vi "Parse Data INSPVAX(SubVI).vi"(11 "Parse Data Array":string[](array[string])=["37.37010082408", "126.72084278410", "9.8363", "22.3000", "-0.0077", "0.0002", "0.0002", "-0.786930858", "0.220983047", "80.255496235", "0.2109", "0.1616", "0.2842", "0.0344", "0.0343", "0.0312", "0.0727", "0.0733", "4.8905", "0f000005", "0*84218c18\n\t"]) -> (3 "output cluster":T1={"Latitude"={"Valid?"=TRUE, "Latitude (Deg)"=37.37010082408}, "Longitude"={"Valid?"=TRUE, "Longitude (Deg)"=126.7208427841}, "Height"={"Valid?"=TRUE, "Height (m)"=9.8363}, "Undulation"={"Valid?"=TRUE, "Undulation(m)"=22.3}, "North Vel"={"Valid?"=TRUE, "North Vel (m/s)"=-0.0077}, "East Vel"={"Valid?"=TRUE, "East Vel (m/s)"=0.0002}, "Up Vel"={"Valid?"=TRUE, "Up Vel (m/s)"=0.0002}, "Roll"={"Valid?"=TRUE, "Roll (degrees)"=-0.786930858}, "Pitch"={"Valid?"=TRUE, "Pitch (degrees)"=0.220983047}, "Azimuth"={"Valid?"=TRUE, "Azimuth (degrees)"=80.255496235}, "Lat deviation"={"Valid?"=TRUE, "Lat deviation (m)"=0.2109}, "Long deviation"={"Valid?"=TRUE, "Long deviation (m)"=0.1616}, "Height deviation"={"Valid?"=TRUE, "Height deviation (m)"=0.2842}, "North vel deviation"={"Valid?"=TRUE, "North vel deviation (m/s)"=0.0344}, "East vel deviation"={"Valid?"=TRUE, "East vel deviation (m/s)"=0.0343}, "Up vel deviation"={"Valid?"=TRUE, "Up vel deviation (m/s)"=0.0312}, "Roll deviation"={"Valid?"=TRUE, "Roll deviation (degrees)"=0.0727}, "Pitch deviation"={"Valid?"=TRUE, "Pitch deviation (degrees)"=0.0733}, "Azimuth deviation"={"Valid?"=TRUE, "Azimuth deviation (degrees)"=4.8905}, "Ext sol status"={"Valid?"=TRUE, "Ext sol status"=0.0}})   [LabVIEW 2019]
panel:
  out "x = y?":bool=TRUE
  out "size":i32=21
  out "output cluster 2":T1={"Latitude"={"Valid?"=TRUE, "Latitude (Deg)"=37.37010082408}, "Longitude"={"Valid?"=TRUE, "Longitude (Deg)"=126.7208427841}, "Height"={"Valid?"=TRUE, "Height (m)"=9.8363}, "Undulation"={"Valid?"=TRUE, "Undulation(m)"=22.3}, "North Vel"={"Valid?"=TRUE, "North Vel (m/s)"=-0.0077}, "East Vel"={"Valid?"=TRUE, "East Vel (m/s)"=0.0002}, "Up Vel"={"Valid?"=TRUE, "Up Vel (m/s)"=0.0002}, "Roll"={"Valid?"=TRUE, "Roll (degrees)"=-0.786930858}, "Pitch"={"Valid?"=TRUE, "Pitch (degrees)"=0.220983047}, "Azimuth"={"Valid?"=TRUE, "Azimuth (degrees)"=80.255496235}, "Lat deviation"={"Valid?"=TRUE, "Lat deviation (m)"=0.2109}, "Long deviation"={"Valid?"=TRUE, "Long deviation (m)"=0.1616}, "Height deviation"={"Valid?"=TRUE, "Height deviation (m)"=0.2842}, "North vel deviation"={"Valid?"=TRUE, "North vel deviation (m/s)"=0.0344}, "East vel deviation"={"Valid?"=TRUE, "East vel deviation (m/s)"=0.0343}, "Up vel deviation"={"Valid?"=TRUE, "Up vel deviation (m/s)"=0.0312}, "Roll deviation"={"Valid?"=TRUE, "Roll deviation (degrees)"=0.0727}, "Pitch deviation"={"Valid?"=TRUE, "Pitch deviation (degrees)"=0.0733}, "Azimuth deviation"={"Valid?"=TRUE, "Azimuth deviation (degrees)"=4.8905}, "Ext sol status"={"Valid?"=TRUE, "Ext sol status"=0.0}}
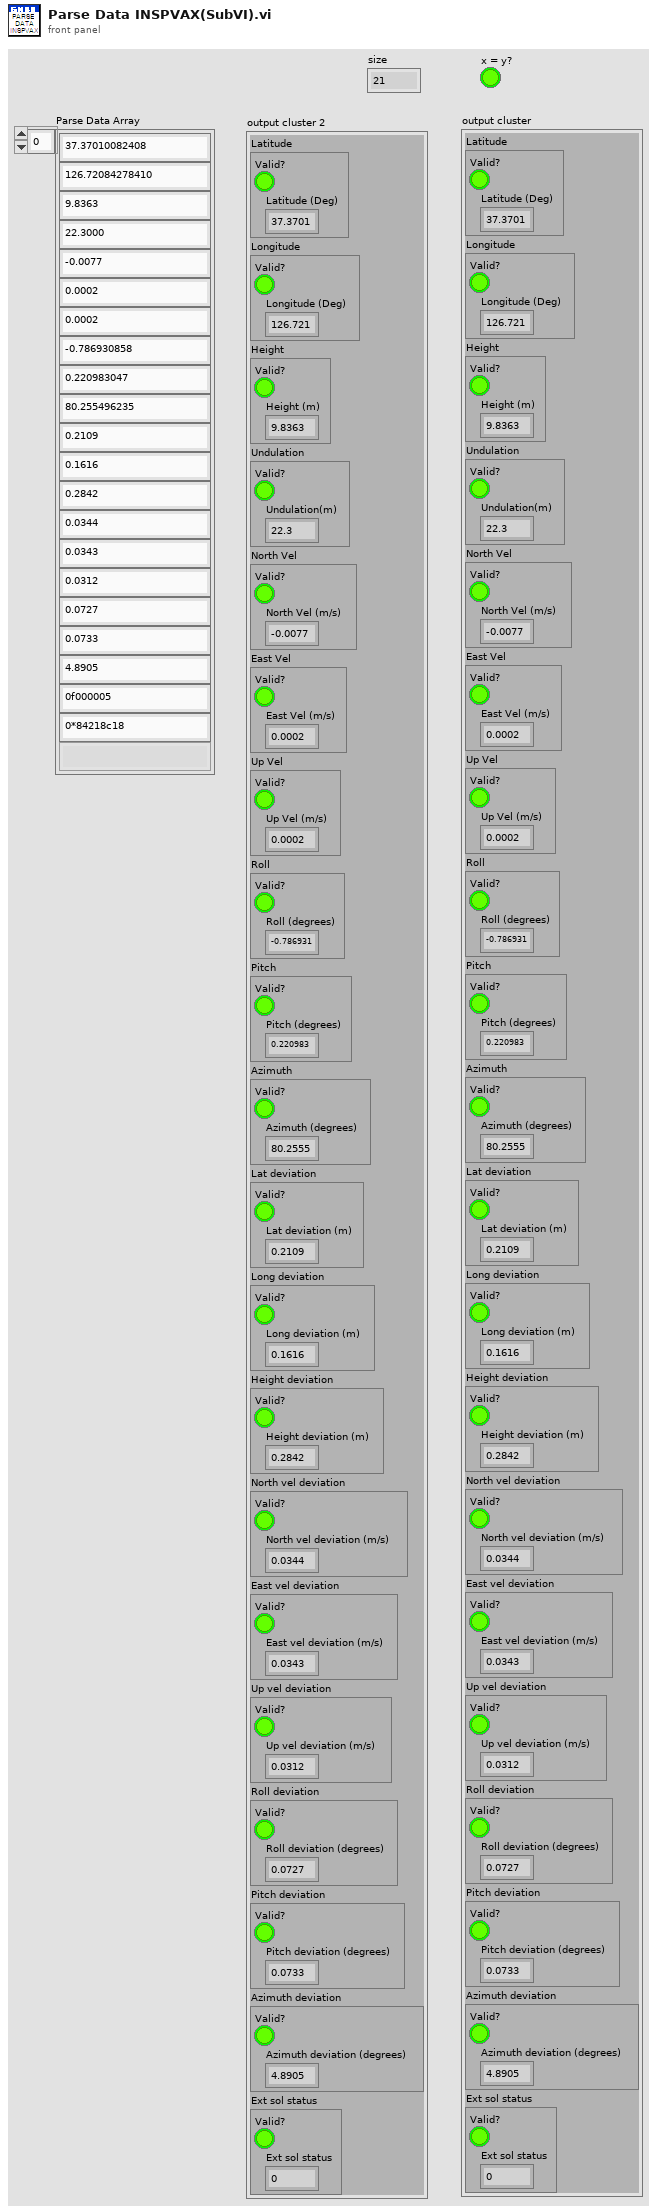
[diagram p1: front panel]
types:
  T1 = cluster{"Latitude":cluster{"Valid?":bool, "Latitude (Deg)":dbl}, "Longitude":cluster{"Valid?":bool, "Longitude (Deg)":dbl}, "Height":cluster{"Valid?":bool, "Height (m)":dbl}, "Undulation":cluster{"Valid?":bool, "Undulation(m)":dbl}, "North Vel":cluster{"Valid?":bool, "North Vel (m/s)":dbl}, "East Vel":cluster{"Valid?":bool, "East Vel (m/s)":dbl}, "Up Vel":cluster{"Valid?":bool, "Up Vel (m/s)":dbl}, "Roll":cluster{"Valid?":bool, "Roll (degrees)":dbl}, "Pitch":cluster{"Valid?":bool, "Pitch (degrees)":dbl}, "Azimuth":cluster{"Valid?":bool, "Azimuth (degrees)":dbl}, "Lat deviation":cluster{"Valid?":bool, "Lat deviation (m)":dbl}, "Long deviation":cluster{"Valid?":bool, "Long deviation (m)":dbl}, "Height deviation":cluster{"Valid?":bool, "Height deviation (m)":dbl}, "North vel deviation":cluster{"Valid?":bool, "North vel deviation (m/s)":dbl}, "East vel deviation":cluster{"Valid?":bool, "East vel deviation (m/s)":dbl}, "Up vel deviation":cluster{"Valid?":bool, "Up vel deviation (m/s)":dbl}, "Roll deviation":cluster{"Valid?":bool, "Roll deviation (degrees)":dbl}, "Pitch deviation":cluster{"Valid?":bool, "Pitch deviation (degrees)":dbl}, "Azimuth deviation":cluster{"Valid?":bool, "Azimuth deviation (degrees)":dbl}, "Ext sol status":cluster{"Valid?":bool, "Ext sol status":dbl}}
  T2 = cluster{"Valid?":bool, "Pitch deviation (degrees)":dbl}
  T3 = cluster{"Valid?":bool, "Azimuth deviation (degrees)":dbl}
  T4 = cluster{"Valid?":bool, "Roll deviation (degrees)":dbl}
  T5 = cluster{"Valid?":bool, "Up vel deviation (m/s)":dbl}
  T6 = cluster{"Valid?":bool, "Height deviation (m)":dbl}
  T7 = cluster{"Valid?":bool, "North vel deviation (m/s)":dbl}
  T8 = cluster{"Valid?":bool, "East vel deviation (m/s)":dbl}
  T9 = cluster{"[0]":cluster{"Valid?":bool, "Latitude (Deg)":dbl}, "[1]":cluster{"Valid?":bool, "Latitude (Deg)":dbl}, "[2]":cluster{"Valid?":bool, "Latitude (Deg)":dbl}, "[3]":cluster{"Valid?":bool, "Latitude (Deg)":dbl}, "[4]":cluster{"Valid?":bool, "Latitude (Deg)":dbl}, "[5]":cluster{"Valid?":bool, "Latitude (Deg)":dbl}, "[6]":cluster{"Valid?":bool, "Latitude (Deg)":dbl}, "[7]":cluster{"Valid?":bool, "Latitude (Deg)":dbl}, "[8]":cluster{"Valid?":bool, "Latitude (Deg)":dbl}, "[9]":cluster{"Valid?":bool, "Latitude (Deg)":dbl}, "[10]":cluster{"Valid?":bool, "Latitude (Deg)":dbl}, "[11]":cluster{"Valid?":bool, "Latitude (Deg)":dbl}, "[12]":cluster{"Valid?":bool, "Latitude (Deg)":dbl}, "[13]":cluster{"Valid?":bool, "Latitude (Deg)":dbl}, "[14]":cluster{"Valid?":bool, "Latitude (Deg)":dbl}, "[15]":cluster{"Valid?":bool, "Latitude (Deg)":dbl}, "[16]":cluster{"Valid?":bool, "Latitude (Deg)":dbl}, "[17]":cluster{"Valid?":bool, "Latitude (Deg)":dbl}, "[18]":cluster{"Valid?":bool, "Latitude (Deg)":dbl}, "[19]":cluster{"Valid?":bool, "Latitude (Deg)":dbl}}
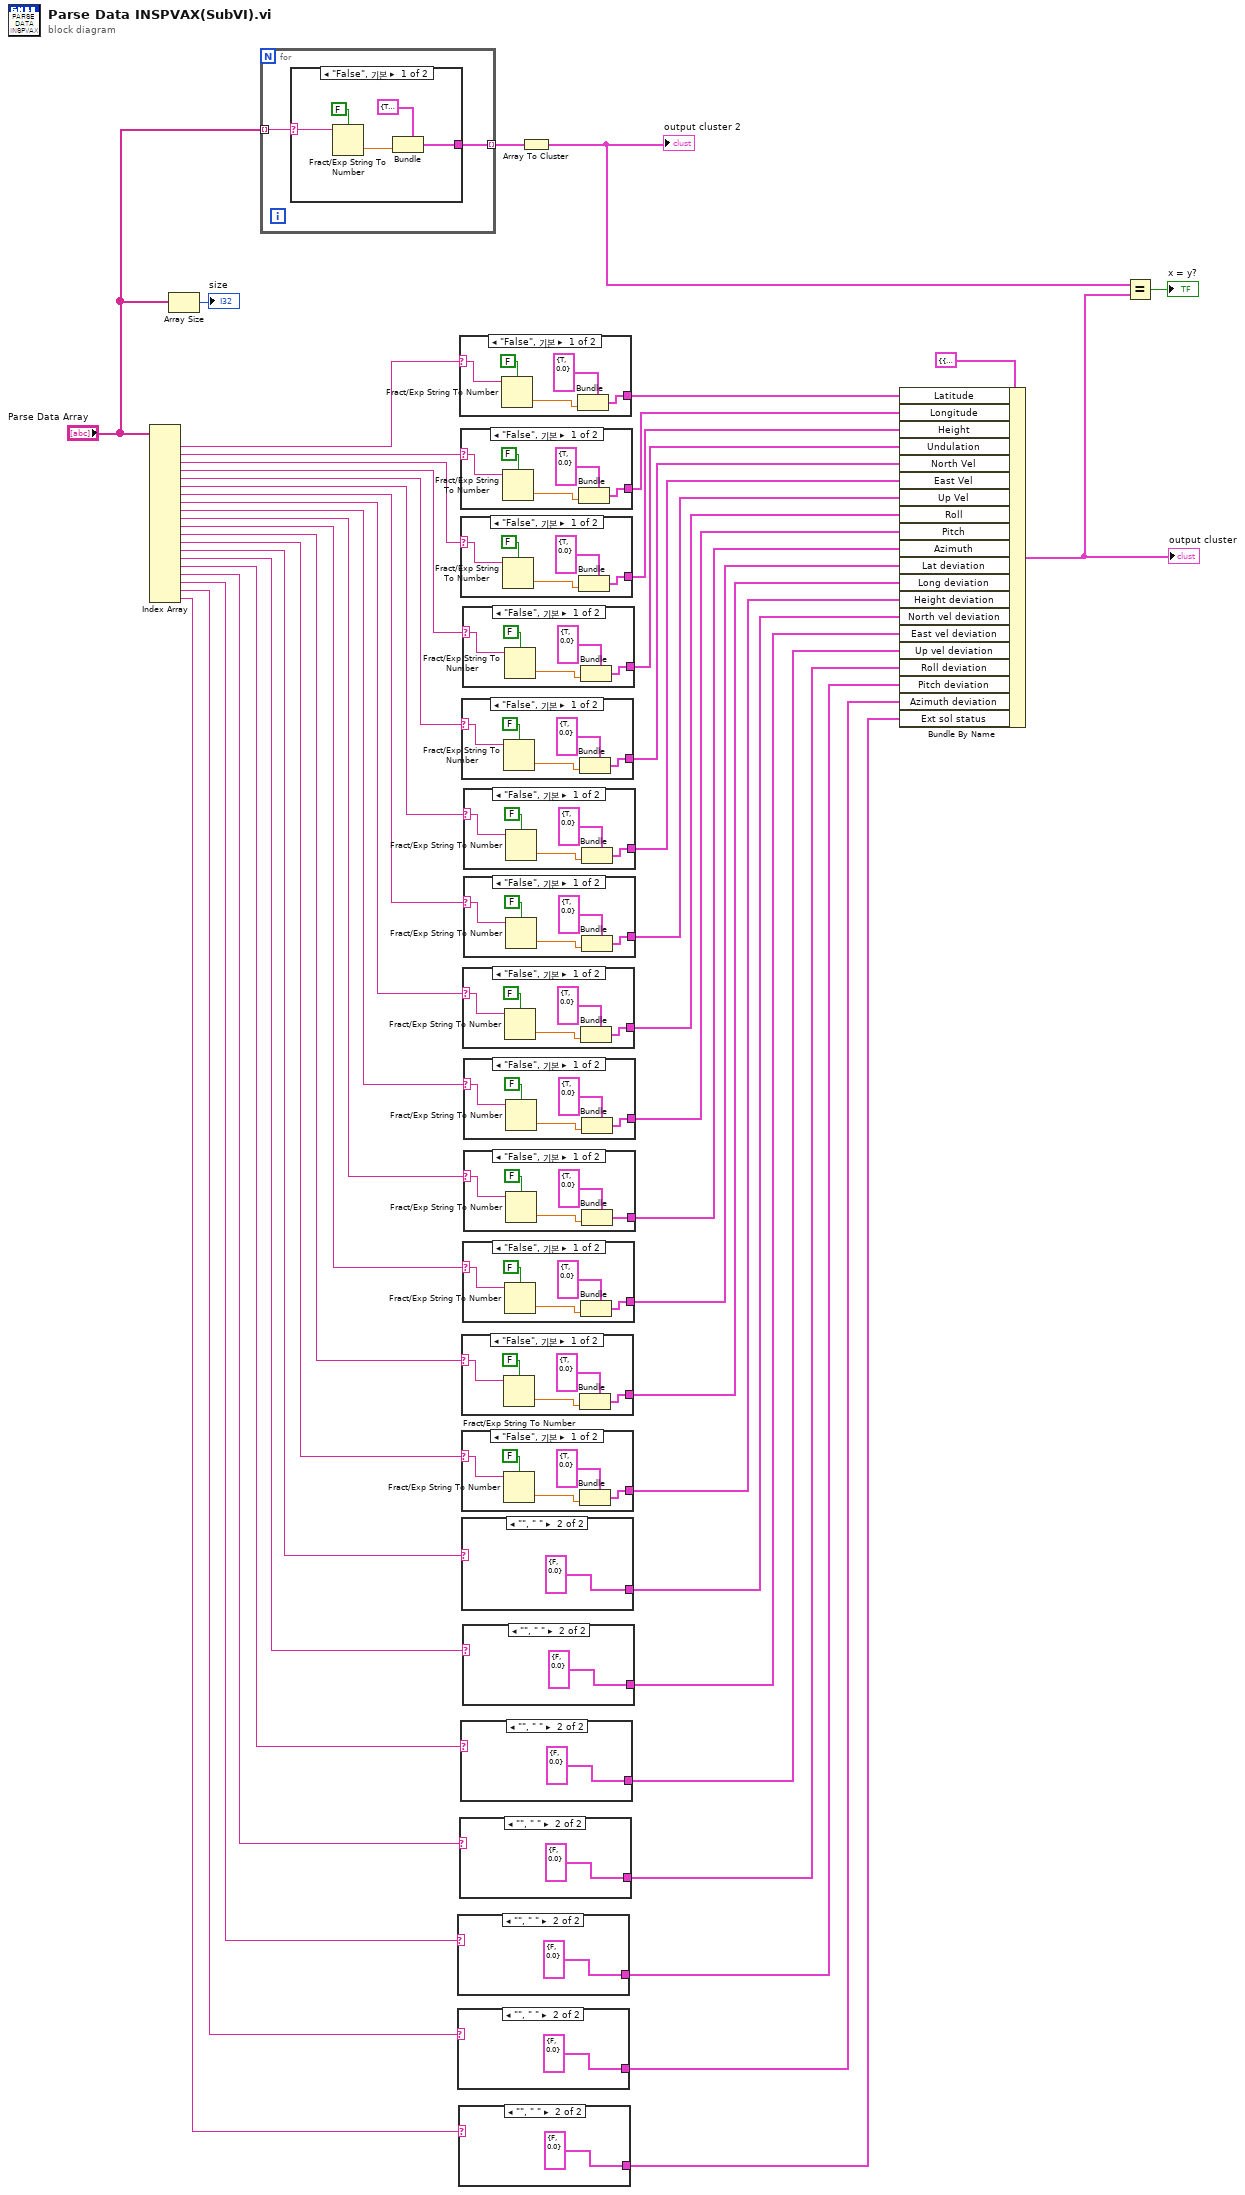
[diagram p0: block diagram]
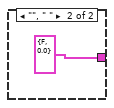
[diagram p2: hidden frame]
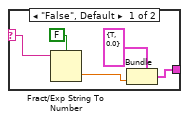
[diagram p3: hidden frame]
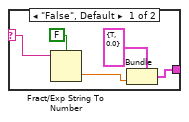
[diagram p4: hidden frame]
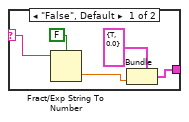
[diagram p5: hidden frame]
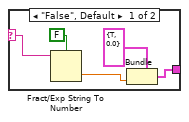
[diagram p6: hidden frame]
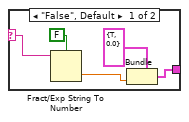
[diagram p7: hidden frame]
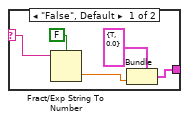
[diagram p8: hidden frame]
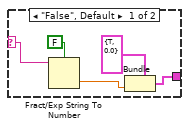
[diagram p9: hidden frame]
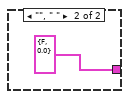
[diagram p10: hidden frame]
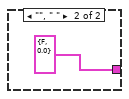
[diagram p11: hidden frame]
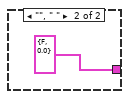
[diagram p12: hidden frame]
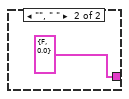
[diagram p13: hidden frame]
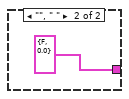
[diagram p14: hidden frame]
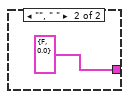
[diagram p15: hidden frame]
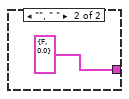
[diagram p16: hidden frame]
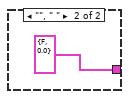
[diagram p17: hidden frame]
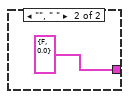
[diagram p18: hidden frame]
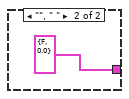
[diagram p19: hidden frame]
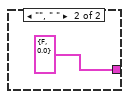
[diagram p20: hidden frame]
diagram:
  n1 = Index Array(array="Parse Data Array") -> (element #1=w47:string, element #2=w46:string, element #3=w45:string, element #4=w44:string, element #5=w43:string, element #6=w42:string, element #7=w41:string, element #8=w40:string, element #9=w39:string, element #10=w38:string, element #11=w37:string, element #12=w36:string, element #13=w35:string, element #14=w34:string, element #15=w33:string, element #16=w32:string, element #17=w31:string, element #18=w30:string, element #19=w29:string, element #20=w28:string)  [unwired: 20 in]
  n2 = Array Size(array="Parse Data Array") -> (size(s)=→"size":i32)
  n3 = for {
    tunnel: "Parse Data Array" -> [w49] mode=indexing
    tunnel: [w48] -> w6 mode=indexing
    n4 = case shown="\"False\", 기본" w49 {
      selector: w49 -> [w53 _]
      tunnel: [w50 cluster{"Valid?":bool, "Latitude (Deg)":dbl} {"Valid?"=FALSE, "Latitude (Deg)"=0.0} ("Latitude")] -> w48
      frame "False", Default {
        n5 = Fract/Exp String To Number(use system decimal point (T)=FALSE, string=w53) -> (number=w54:dbl)  [unwired: 3 out]
        n6 = Bundle(cluster=cluster{"Valid?":bool, "Latitude (Deg)":dbl} {"Valid?"=TRUE, "Latitude (Deg)"=0.0} ("Latitude"), "Latitude (Deg)"=w54) -> (w50:cluster{"Valid?":bool, "Latitude (Deg)":dbl})  [unwired: 1 out]
      }
      frame "", " " {
      }
    }
  }
  n7 = case shown="\"\", \" \"" w30 {
    selector: w30 -> [w59 _]
    tunnel: [w57 T2 {"Valid?"=FALSE, "Pitch deviation (degrees)"=0.0} ("Pitch deviation")] -> w9
    frame "False", Default {
      n8 = Fract/Exp String To Number(use system decimal point (T)=FALSE, string=w59) -> (number=w60:dbl)  [unwired: 3 out]
      n9 = Bundle(cluster=T2 {"Valid?"=TRUE, "Pitch deviation (degrees)"=0.0} ("Pitch deviation"), "Pitch deviation (degrees)"=w60) -> (w57:T2)  [unwired: 1 out]
    }
    frame "", " " {
    }
  }
  n10 = case shown="\"\", \" \"" w29 {
    selector: w29 -> [w65 _]
    tunnel: [w63 T3 {"Valid?"=FALSE, "Azimuth deviation (degrees)"=0.0} ("Azimuth deviation")] -> w8
    frame "False", Default {
      n11 = Fract/Exp String To Number(use system decimal point (T)=FALSE, string=w65) -> (number=w66:dbl)  [unwired: 3 out]
      n12 = Bundle(cluster=T3 {"Valid?"=TRUE, "Azimuth deviation (degrees)"=0.0} ("Azimuth deviation"), "Azimuth deviation (degrees)"=w66) -> (w63:T3)  [unwired: 1 out]
    }
    frame "", " " {
    }
  }
  n13 = case shown="\"\", \" \"" w28 {
    selector: w28 -> [w71 _]
    tunnel: [w69 cluster{"Valid?":bool, "Ext sol status":dbl} {"Valid?"=FALSE, "Ext sol status"=0.0} ("Ext sol status")] -> w7
    frame "False", Default {
      n14 = Fract/Exp String To Number(use system decimal point (T)=FALSE, string=w71) -> (number=w72:dbl)  [unwired: 3 out]
      n15 = Bundle(cluster=cluster{"Valid?":bool, "Ext sol status":dbl} {"Valid?"=TRUE, "Ext sol status"=0.0} ("Ext sol status"), "Ext sol status"=w72) -> (w69:cluster{"Valid?":bool, "Ext sol status":dbl})  [unwired: 1 out]
    }
    frame "", " " {
    }
  }
  n16 = case shown="\"False\", 기본" w47 {
    selector: w47 -> [w77 _]
    tunnel: [w74 cluster{"Valid?":bool, "Latitude (Deg)":dbl} {"Valid?"=FALSE, "Latitude (Deg)"=0.0} ("Latitude")] -> w26
    frame "False", Default {
      n17 = Fract/Exp String To Number(use system decimal point (T)=FALSE, string=w77) -> (number=w78:dbl)  [unwired: 3 out]
      n18 = Bundle(cluster=cluster{"Valid?":bool, "Latitude (Deg)":dbl} {"Valid?"=TRUE, "Latitude (Deg)"=0.0} ("Latitude"), "Latitude (Deg)"=w78) -> (w74:cluster{"Valid?":bool, "Latitude (Deg)":dbl})  [unwired: 1 out]
    }
    frame "", " " {
    }
  }
  n19 = case shown="\"\", \" \"" w31 {
    selector: w31 -> [w83 _]
    tunnel: [w81 T4 {"Valid?"=FALSE, "Roll deviation (degrees)"=0.0} ("Roll deviation")] -> w10
    frame "False", Default {
      n20 = Fract/Exp String To Number(use system decimal point (T)=FALSE, string=w83) -> (number=w84:dbl)  [unwired: 3 out]
      n21 = Bundle(cluster=T4 {"Valid?"=TRUE, "Roll deviation (degrees)"=0.0} ("Roll deviation"), "Roll deviation (degrees)"=w84) -> (w81:T4)  [unwired: 1 out]
    }
    frame "", " " {
    }
  }
  n22 = case shown="\"False\", 기본" w46 {
    selector: w46 -> [w89 _]
    tunnel: [w87 cluster{"Valid?":bool, "Longitude (Deg)":dbl} {"Valid?"=FALSE, "Longitude (Deg)"=0.0} ("Longitude")] -> w25
    frame "False", Default {
      n23 = Fract/Exp String To Number(use system decimal point (T)=FALSE, string=w89) -> (number=w90:dbl)  [unwired: 3 out]
      n24 = Bundle(cluster=cluster{"Valid?":bool, "Longitude (Deg)":dbl} {"Valid?"=TRUE, "Longitude (Deg)"=0.0} ("Longitude"), "Longitude (Deg)"=w90) -> (w87:cluster{"Valid?":bool, "Longitude (Deg)":dbl})  [unwired: 1 out]
    }
    frame "", " " {
    }
  }
  n25 = case shown="\"False\", 기본" w45 {
    selector: w45 -> [w95 _]
    tunnel: [w93 cluster{"Valid?":bool, "Height(m)":dbl} {"Valid?"=FALSE, "Height(m)"=0.0} ("Height")] -> w24
    frame "False", Default {
      n26 = Fract/Exp String To Number(use system decimal point (T)=FALSE, string=w95) -> (number=w96:dbl)  [unwired: 3 out]
      n27 = Bundle(cluster=cluster{"Valid?":bool, "Height(m)":dbl} {"Valid?"=TRUE, "Height(m)"=0.0} ("Height\nHeight"), "Height(m)"=w96) -> (w93:cluster{"Valid?":bool, "Height(m)":dbl})  [unwired: 1 out]
    }
    frame "", " " {
    }
  }
  n28 = case shown="\"\", \" \"" w32 {
    selector: w32 -> [w101 _]
    tunnel: [w99 T5 {"Valid?"=FALSE, "Up vel deviation (m/s)"=0.0} ("Up vel deviation")] -> w11
    frame "False", Default {
      n29 = Fract/Exp String To Number(use system decimal point (T)=FALSE, string=w101) -> (number=w102:dbl)  [unwired: 3 out]
      n30 = Bundle(cluster=T5 {"Valid?"=TRUE, "Up vel deviation (m/s)"=0.0} ("Up vel deviation"), "Up vel deviation (m/s)"=w102) -> (w99:T5)  [unwired: 1 out]
    }
    frame "", " " {
    }
  }
  n31 = case shown="\"False\", 기본" w43 {
    selector: w43 -> [w107 _]
    tunnel: [w105 cluster{"Valid?":bool, "North Vel (m/s)":dbl} {"Valid?"=FALSE, "North Vel (m/s)"=0.0} ("North Vel")] -> w22
    frame "False", Default {
      n32 = Fract/Exp String To Number(use system decimal point (T)=FALSE, string=w107) -> (number=w108:dbl)  [unwired: 3 out]
      n33 = Bundle(cluster=cluster{"Valid?":bool, "North Vel (m/s)":dbl} {"Valid?"=TRUE, "North Vel (m/s)"=0.0} ("North Vel"), "North Vel (m/s)"=w108) -> (w105:cluster{"Valid?":bool, "North Vel (m/s)":dbl})  [unwired: 1 out]
    }
    frame "", " " {
    }
  }
  n34 = case shown="\"False\", 기본" w36 {
    selector: w36 -> [w113 _]
    tunnel: [w111 cluster{"Valid?":bool, "Long deviation (m)":dbl} {"Valid?"=FALSE, "Long deviation (m)"=0.0} ("Long deviation")] -> w15
    frame "False", Default {
      n35 = Fract/Exp String To Number(use system decimal point (T)=FALSE, string=w113) -> (number=w114:dbl)  [unwired: 3 out]
      n36 = Bundle(cluster=cluster{"Valid?":bool, "Long deviation (m)":dbl} {"Valid?"=TRUE, "Long deviation (m)"=0.0} ("Long deviation"), "Long deviation (m)"=w114) -> (w111:cluster{"Valid?":bool, "Long deviation (m)":dbl})  [unwired: 1 out]
    }
    frame "", " " {
    }
  }
  n37 = case shown="\"False\", 기본" w35 {
    selector: w35 -> [w119 _]
    tunnel: [w117 T6 {"Valid?"=FALSE, "Height deviation (m)"=0.0} ("Height deviation")] -> w14
    frame "False", Default {
      n38 = Fract/Exp String To Number(use system decimal point (T)=FALSE, string=w119) -> (number=w120:dbl)  [unwired: 3 out]
      n39 = Bundle(cluster=T6 {"Valid?"=TRUE, "Height deviation (m)"=0.0} ("Height deviation"), "Height deviation (m)"=w120) -> (w117:T6)  [unwired: 1 out]
    }
    frame "", " " {
    }
  }
  n40 = case shown="\"\", \" \"" w34 {
    selector: w34 -> [w125 _]
    tunnel: [w123 T7 {"Valid?"=FALSE, "North vel deviation (m/s)"=0.0} ("North vel deviation")] -> w13
    frame "False", Default {
      n41 = Fract/Exp String To Number(use system decimal point (T)=FALSE, string=w125) -> (number=w126:dbl)  [unwired: 3 out]
      n42 = Bundle(cluster=T7 {"Valid?"=TRUE, "North vel deviation (m/s)"=0.0} ("Long deviation"), "North vel deviation (m/s)"=w126) -> (w123:T7)  [unwired: 1 out]
    }
    frame "", " " {
    }
  }
  n43 = case shown="\"False\", 기본" w44 {
    selector: w44 -> [w131 _]
    tunnel: [w129 cluster{"Valid?":bool, "Undulation (m)":dbl} {"Valid?"=FALSE, "Undulation (m)"=0.0} ("Undulation")] -> w23
    frame "False", Default {
      n44 = Fract/Exp String To Number(use system decimal point (T)=FALSE, string=w131) -> (number=w132:dbl)  [unwired: 3 out]
      n45 = Bundle(cluster=cluster{"Valid?":bool, "Undulation (m)":dbl} {"Valid?"=TRUE, "Undulation (m)"=0.0} ("Undulation"), "Undulation (m)"=w132) -> (w129:cluster{"Valid?":bool, "Undulation (m)":dbl})  [unwired: 1 out]
    }
    frame "", " " {
    }
  }
  n46 = case shown="\"False\", 기본" w40 {
    selector: w40 -> [w137 _]
    tunnel: [w135 cluster{"Valid?":bool, "Roll (degrees)":dbl} {"Valid?"=FALSE, "Roll (degrees)"=0.0} ("Roll")] -> w19
    frame "False", Default {
      n47 = Fract/Exp String To Number(use system decimal point (T)=FALSE, string=w137) -> (number=w138:dbl)  [unwired: 3 out]
      n48 = Bundle(cluster=cluster{"Valid?":bool, "Roll (degrees)":dbl} {"Valid?"=TRUE, "Roll (degrees)"=0.0} ("Roll"), "Roll (degrees)"=w138) -> (w135:cluster{"Valid?":bool, "Roll (degrees)":dbl})  [unwired: 1 out]
    }
    frame "", " " {
    }
  }
  n49 = case shown="\"False\", 기본" w37 {
    selector: w37 -> [w143 _]
    tunnel: [w141 cluster{"Valid?":bool, "Lat deviation (m)":dbl} {"Valid?"=FALSE, "Lat deviation (m)"=0.0} ("Lat deviation")] -> w16
    frame "False", Default {
      n50 = Fract/Exp String To Number(use system decimal point (T)=FALSE, string=w143) -> (number=w144:dbl)  [unwired: 3 out]
      n51 = Bundle(cluster=cluster{"Valid?":bool, "Lat deviation (m)":dbl} {"Valid?"=TRUE, "Lat deviation (m)"=0.0} ("Lat deviation"), "Lat deviation (m)"=w144) -> (w141:cluster{"Valid?":bool, "Lat deviation (m)":dbl})  [unwired: 1 out]
    }
    frame "", " " {
    }
  }
  n52 = case shown="\"\", \" \"" w33 {
    selector: w33 -> [w149 _]
    tunnel: [w147 T8 {"Valid?"=FALSE, "East vel deviation (m/s)"=0.0} ("East vel deviation")] -> w12
    frame "False", Default {
      n53 = Fract/Exp String To Number(use system decimal point (T)=FALSE, string=w149) -> (number=w150:dbl)  [unwired: 3 out]
      n54 = Bundle(cluster=T8 {"Valid?"=TRUE, "East vel deviation (m/s)"=0.0} ("East vel deviation"), "East vel deviation (m/s)"=w150) -> (w147:T8)  [unwired: 1 out]
    }
    frame "", " " {
    }
  }
  n55 = case shown="\"False\", 기본" w42 {
    selector: w42 -> [w155 _]
    tunnel: [w153 cluster{"Valid?":bool, "East Vel (m/s)":dbl} {"Valid?"=FALSE, "East Vel (m/s)"=0.0} ("East Vel")] -> w21
    frame "False", Default {
      n56 = Fract/Exp String To Number(use system decimal point (T)=FALSE, string=w155) -> (number=w156:dbl)  [unwired: 3 out]
      n57 = Bundle(cluster=cluster{"Valid?":bool, "East Vel (m/s)":dbl} {"Valid?"=TRUE, "East Vel (m/s)"=0.0} ("East Vel"), "East Vel (m/s)"=w156) -> (w153:cluster{"Valid?":bool, "East Vel (m/s)":dbl})  [unwired: 1 out]
    }
    frame "", " " {
    }
  }
  n58 = case shown="\"False\", 기본" w41 {
    selector: w41 -> [w161 _]
    tunnel: [w159 cluster{"Valid?":bool, "Up Vel (m/s)":dbl} {"Valid?"=FALSE, "Up Vel (m/s)"=0.0} ("Up Vel")] -> w20
    frame "False", Default {
      n59 = Fract/Exp String To Number(use system decimal point (T)=FALSE, string=w161) -> (number=w162:dbl)  [unwired: 3 out]
      n60 = Bundle(cluster=cluster{"Valid?":bool, "Up Vel (m/s)":dbl} {"Valid?"=TRUE, "Up Vel (m/s)"=0.0} ("Up Vel"), "Up Vel (m/s)"=w162) -> (w159:cluster{"Valid?":bool, "Up Vel (m/s)":dbl})  [unwired: 1 out]
    }
    frame "", " " {
    }
  }
  n61 = case shown="\"False\", 기본" w39 {
    selector: w39 -> [w167 _]
    tunnel: [w165 cluster{"Valid?":bool, "Pitch (degrees)":dbl} {"Valid?"=FALSE, "Pitch (degrees)"=0.0} ("Pitch")] -> w18
    frame "False", Default {
      n62 = Fract/Exp String To Number(use system decimal point (T)=FALSE, string=w167) -> (number=w168:dbl)  [unwired: 3 out]
      n63 = Bundle(cluster=cluster{"Valid?":bool, "Pitch (degrees)":dbl} {"Valid?"=TRUE, "Pitch (degrees)"=0.0} ("Ritch"), "Pitch (degrees)"=w168) -> (w165:cluster{"Valid?":bool, "Pitch (degrees)":dbl})  [unwired: 1 out]
    }
    frame "", " " {
    }
  }
  n64 = case shown="\"False\", 기본" w38 {
    selector: w38 -> [w173 _]
    tunnel: [w170 cluster{"Valid?":bool, "Azimuth (degrees)":dbl} {"Valid?"=FALSE, "Azimuth (degrees)"=0.0} ("Azimuth")] -> w17
    frame "False", Default {
      n65 = Fract/Exp String To Number(use system decimal point (T)=FALSE, string=w173) -> (number=w174:dbl)  [unwired: 3 out]
      n66 = Bundle(cluster=cluster{"Valid?":bool, "Azimuth (degrees)":dbl} {"Valid?"=TRUE, "Azimuth (degrees)"=0.0} ("Azimuth"), "Azimuth (degrees)"=w174) -> (w170:cluster{"Valid?":bool, "Azimuth (degrees)":dbl})  [unwired: 1 out]
    }
    frame "", " " {
    }
  }
  n67 = Array To Cluster(array=w6) -> (cluster=w2:T9)
  "output cluster 2" <- w2
  n68 = Bundle By Name(cluster=T1 {"Latitude"={"Valid?"=FALSE, "Latitude (Deg)"=0.0}, "Longitude"={"Valid?"=FALSE, "Longitude (Deg)"=0.0}, "Height"={"Valid?"=FALSE, "Height (m)"=0.0}, "Undulation"={"Valid?"=FALSE, "Undulation(m)"=0.0}, "North Vel"={"Valid?"=FALSE, "North Vel (m/s)"=0.0}, "East Vel"={"Valid?"=FALSE, "East Vel (m/s)"=0.0}, "Up Vel"={"Valid?"=FALSE, "Up Vel (m/s)"=0.0}, "Roll"={"Valid?"=FALSE, "Roll (degrees)"=0.0}, "Pitch"={"Valid?"=FALSE, "Pitch (degrees)"=0.0}, "Azimuth"={"Valid?"=FALSE, "Azimuth (degrees)"=0.0}, "Lat deviation"={"Valid?"=FALSE, "Lat deviation (m)"=0.0}, "Long deviation"={"Valid?"=FALSE, "Long deviation (m)"=0.0}, "Height deviation"={"Valid?"=FALSE, "Height deviation (m)"=0.0}, "North vel deviation"={"Valid?"=FALSE, "North vel deviation (m/s)"=0.0}, "East vel deviation"={"Valid?"=FALSE, "East vel deviation (m/s)"=0.0}, "Up vel deviation"={"Valid?"=FALSE, "Up vel deviation (m/s)"=0.0}, "Roll deviation"={"Valid?"=FALSE, "Roll deviation (degrees)"=0.0}, "Pitch deviation"={"Valid?"=FALSE, "Pitch deviation (degrees)"=0.0}, "Azimuth deviation"={"Valid?"=FALSE, "Azimuth deviation (degrees)"=0.0}, "Ext sol status"={"Valid?"=FALSE, "Ext sol status"=0.0}}, "Latitude"=w26, "Longitude"=w25, "Height"=w24, "Undulation"=w23, "North Vel"=w22, "East Vel"=w21, "Up Vel"=w20, "Roll"=w19, "Pitch"=w18, "Azimuth"=w17, "Lat deviation"=w16, "Long deviation"=w15, "Height deviation"=w14, "North vel deviation"=w13, "East vel deviation"=w12, "Up vel deviation"=w11, "Roll deviation"=w10, "Pitch deviation"=w9, "Azimuth deviation"=w8, "Ext sol status"=w7) -> (w3:T1)
  "output cluster" <- w3
  n69 = Equal?(x=w2, y=w3) -> (x = y?=→"x = y?":bool)
